vi "update_currents_test.vi"() -> ()   [LabVIEW 2011]
uses:
  2 Typedefs/Velocity.ctl
  2 Typedefs/heading.ctl
  2 Globals/2 Global.vi
panel:
  in  "stop":bool
  out "x*y":T1 format="%05.1f"
  in  "Boolean":bool
  out "Current/Drift":T2
  in  "Heading":dbl
  in  "Think Freq":dbl
  in  "North 2":dbl
  in  "East 2":dbl
  in  "North":dbl
  in  "East":dbl
  # "Current Val"
  # "Location"
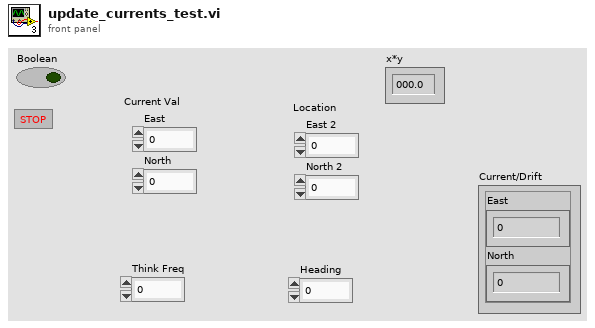
[diagram p1: front panel]
types:
  T1 = typedef "heading.ctl" = dbl
  T2 = typedef "Velocity.ctl" = cluster{"East":dbl, "North":dbl}
  T3 = typedef "UTM Location.ctl" = cluster{"UTM Zone":dbl, "Hemisphere":enum16{"North", "South"}, "East":dbl, "North":dbl}
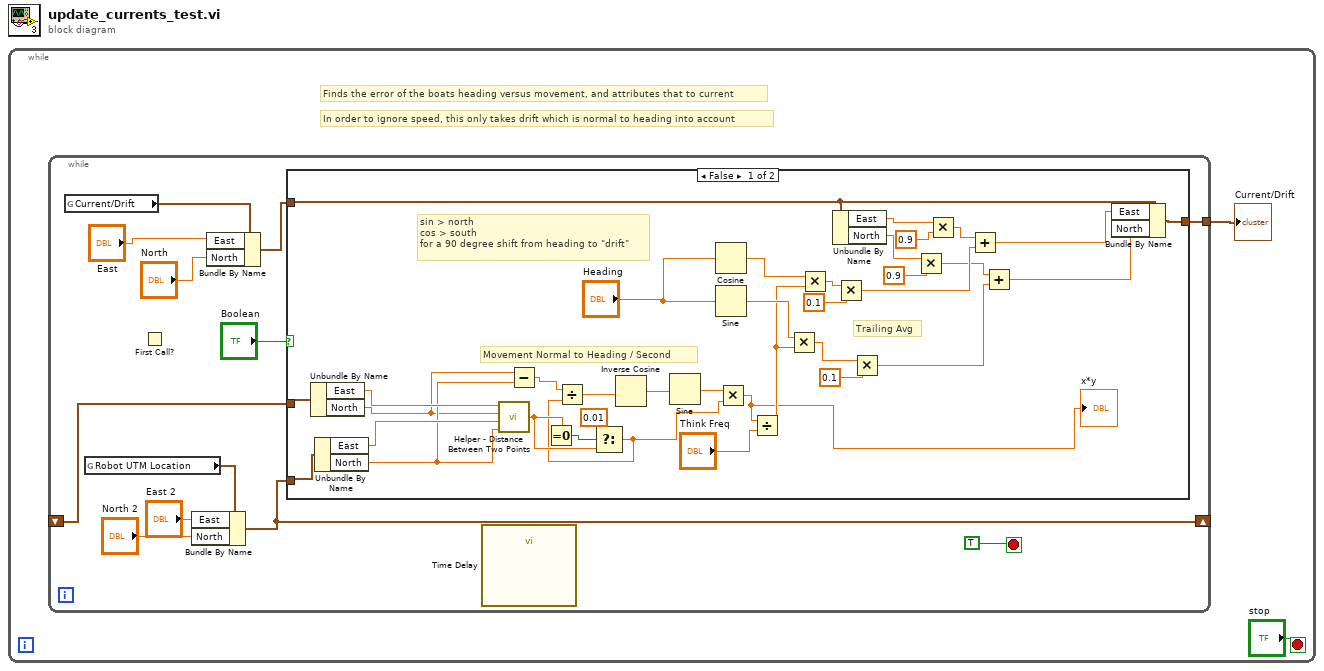
[diagram p0: block diagram]
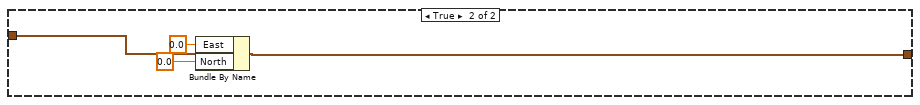
[diagram p2: hidden frame]
diagram:
  n1 = while {
    stop <- "stop" stop-if-true
    # "In order to ignore speed, this only takes drift which is normal to heading into account"
    # "Finds the error of the boats heading versus movement, and attributes that to current"
    n2 = while {
      tunnel: [w14] -> w2
      shift-right: [w8] -> _
      shift-left: _ -> [w12]
      stop <- TRUE stop-if-true
      n3 = global read "2 Global.vi" "Current/Drift"() -> (w11:T2)
      n4 = global read "2 Global.vi" "Robot UTM Location"() -> (w9:T3)
      n5 = First Call?() -> ()  [unwired: 1 out]
      n6 = Bundle By Name(cluster=w9, "East"="East 2", "North"="North 2") -> (w8:T3)
      n7 = Bundle By Name(cluster=w11, "East"="East", "North"="North") -> (w10:T2)
      n8 = case shown="False" "Boolean" {
        tunnel: w10 -> [w39 w54]
        tunnel: [w40 w53] -> w14
        tunnel: w12 -> [w50 _]
        tunnel: w8 -> [w49 _]
        frame False {
          # "Trailing Avg"
          # "sin > north\ncos > south\nfor a 90 degree shift from heading to \"drift\""
          # "Movement Normal to Heading / Second"
          n9 = Unbundle By Name(w50) -> ("East"=w48:dbl, "North"=w45:dbl)
          n10 = Unbundle By Name(w49) -> ("East"=w47:dbl, "North"=w46:dbl)
          n11 = call "Helper - Distance Between Two Points.vi"("y 2"=w46, "x 2"=w47, "y"=w45, "x"=w48) -> ("Numeric"=w19:dbl)
          n12 = Subtract(x=w45, y=w46) -> (x-y=w44:dbl)
          n13 = Equal To 0?(x=w19) -> (x = 0?=w17:bool)
          n14 = Select(t=0.01, s=w17, f=w19) -> (s? t:f=w15:dbl)
          n15 = Divide(x=w44, y=w15) -> (x/y=w43:dbl)
          n16 = Inverse Cosine(1:w43) -> (0:w22:dbl)
          n17 = Sine(x=w22) -> (sin(x)=w21:dbl)
          n18 = Cosine(x="Heading") -> (cos(x)=w41:dbl)
          n19 = Sine(x="Heading") -> (sin(x)=w42:dbl)
          n20 = Multiply(x=w21, y=w15) -> (x*y=w16:dbl)
          "x*y" <- w16
          n21 = Divide(x=w16, y="Think Freq") -> (x/y=w23:dbl)
          n22 = Multiply(x=w42, y=w23) -> (x*y=w35:dbl)
          n23 = Multiply(x=w41, y=w23) -> (x*y=w38:dbl)
          n24 = Unbundle By Name(w39) -> ("East"=w33:dbl, "North"=w31:dbl)
          n25 = Multiply(x=w38, y=T1 0.1) -> (x*y=w29:T1)
          n26 = Multiply(x=w35, y=T1 0.1) -> (x*y=w27:T1)
          n27 = Multiply(x=w31, y=T1 0.9) -> (x*y=w28:T1)
          n28 = Multiply(x=w33, y=T1 0.9) -> (x*y=w30:T1)
          n29 = Add(x=w30, y=w29) -> (x+y=w26:T1)
          n30 = Add(x=w28, y=w27) -> (x+y=w25:T1)
          n31 = Bundle By Name(cluster=w39, "East"=w26, "North"=w25) -> (w40:T2)
        }
        frame True {
          n32 = Bundle By Name(cluster=w54, "East"=0.0, "North"=0.0) -> (w53:T2)
        }
      }
      n33 = call "Time Delay"() -> ()  [unwired: 11 in, 1 out]
    }
    "Current/Drift" <- w2
  }
